vi "Flat.vi"(0 "Vin SMU":refnum<k15>, 1 "Input Voltage":dbl caption="voltage level" format="%.6p", 2 "Load current mA":dbl[](array[numeric]) caption="voltage level" format="%.6p", 5 "Load SMU":refnum<k15>, 7 "Vin DMM":refnum<k15>, 9 "Load DMM":refnum<k15>, 11 "error in (no error)":errorcluster) -> (4 "Load Regulation Ohm":dbl, 6 "Load Regulation %":dbl, 8 "output cluster":T1, 15 "error out":errorcluster)   [LabVIEW 2020]
uses:
  <instrlib>/niDCPower/nidcpower.llb/niDCPower Source Mode.ctl
  <instrlib>/niDCPower/nidcpower.llb/niDCPower Output Function.ctl
panel:
  in  "Nominal Voltage":dbl
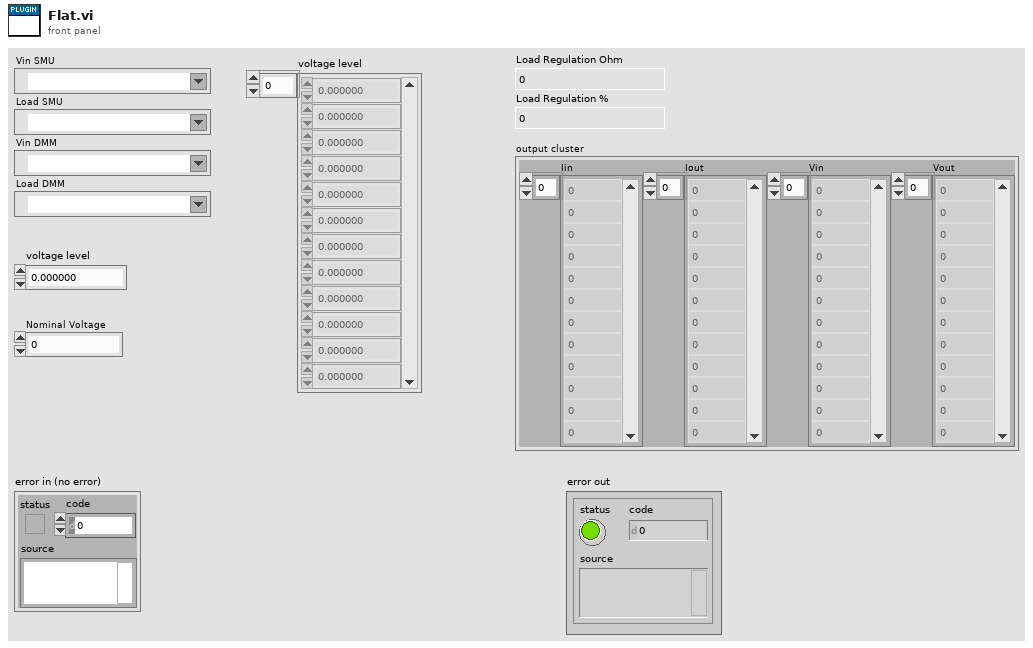
[diagram p1: front panel]
types:
  T1 = cluster{"Iin":dbl[], "Iout":dbl[], "Vin":dbl[], "Vout":dbl[]}
  T2 = typedef "niDCPower Output Function.ctl" = i32
  T3 = typedef "niDCPower Source Mode.ctl" = i32
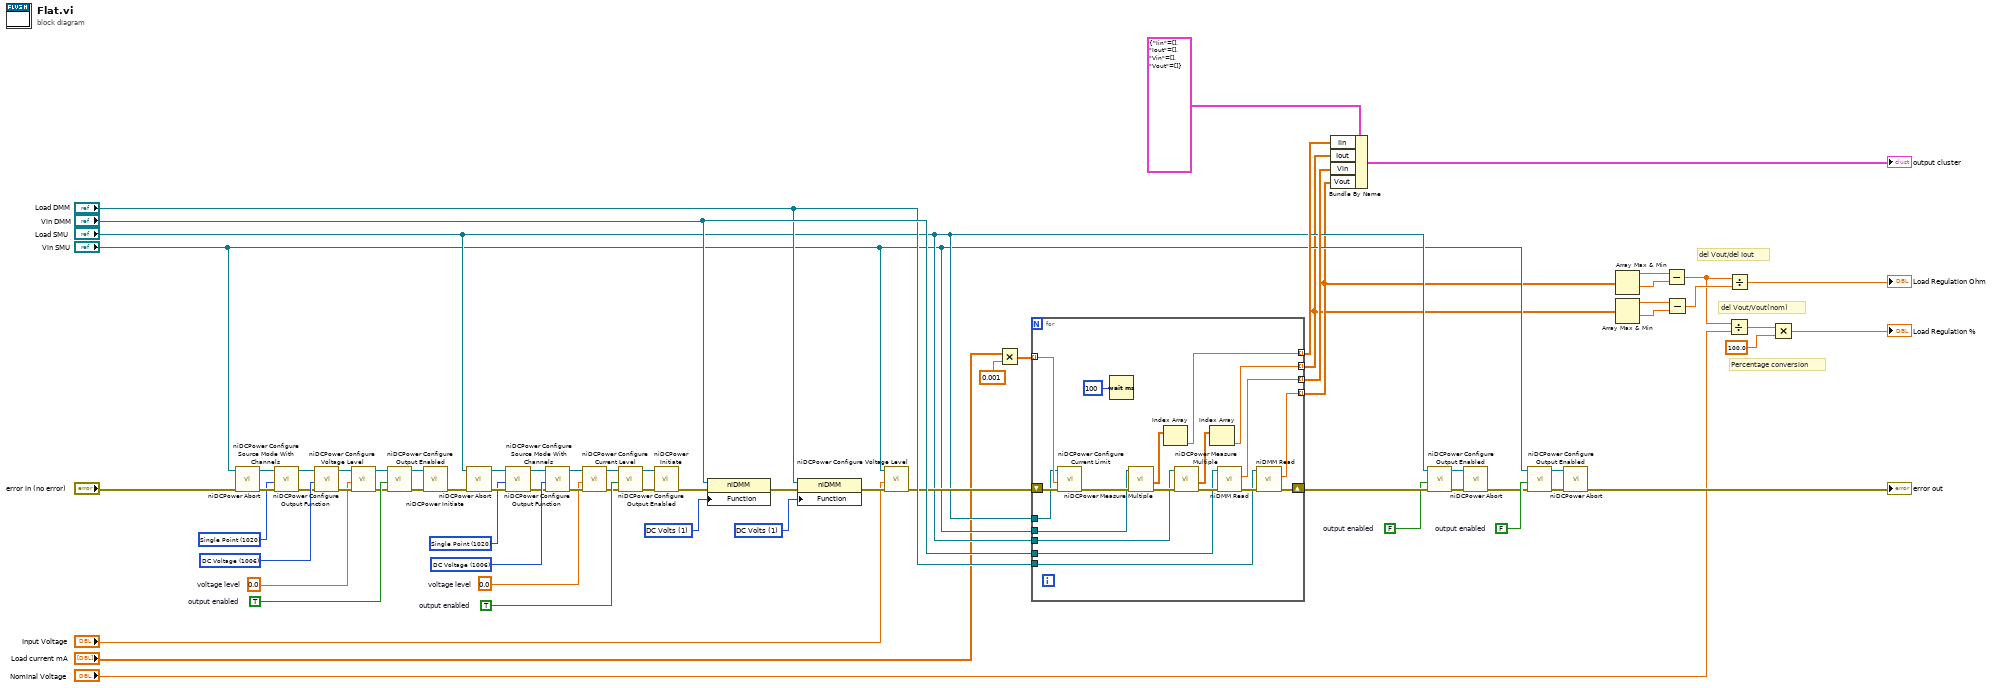
[diagram p0: block diagram]
diagram:
  w25 = FALSE  # output enabled
  w26 = FALSE  # output enabled
  w38 = 1 items=["DC Volts"=1, "AC Volts"=2, "DC Current"=3, "AC Current"=4, "2-Wire Resistance"=5, "4-Wire Resistance"=101, "Frequency"=104, "Period"=105, "AC Volts DC Coupled"=1001, "Diode"=1002, "Waveform Voltage"=1003, "Waveform Current"=1004, "Capacitance"=1005, "Inductance"=1006, "Temperature"=108] ("Configuration:Function")
  w39 = 1 items=["DC Volts"=1, "AC Volts"=2, "DC Current"=3, "AC Current"=4, "2-Wire Resistance"=5, "4-Wire Resistance"=101, "Frequency"=104, "Period"=105, "AC Volts DC Coupled"=1001, "Diode"=1002, "Waveform Voltage"=1003, "Waveform Current"=1004, "Capacitance"=1005, "Inductance"=1006, "Temperature"=108] ("Configuration:Function")
  w43 = 0.0  # voltage level
  w48 = TRUE  # output enabled
  w54 = T2 1006 items=["DC Voltage"=1006, "DC Current"=1007, "Pulse Voltage"=1049, "Pulse Current"=1050] ("output function")
  w51 = T3 1020 items=["Single Point"=1020, "Sequence"=1021] ("source mode")
  w61 = TRUE  # output enabled
  w62 = 0.0  # voltage level
  w68 = T2 1006 items=["DC Voltage"=1006, "DC Current"=1007, "Pulse Voltage"=1049, "Pulse Current"=1050] ("output function")
  w65 = T3 1020 items=["Single Point"=1020, "Sequence"=1021] ("source mode")
  # "del Vout/Vout(nom)"
  # "del Vout/del Iout"
  # "Percentage conversion"
  n1 = call <instrlib>:"niDCPower Abort.vi"("error in (no error)"="error in (no error)", "instrument handle"="Vin SMU") -> ("error out"=w69:errorcluster, "instrument handle out"=w70:refnum<k15>)  [unwired: 8 in]
  n2 = call <instrlib>:"niDCPower Configure Source Mode With Channels.vi"("error in (no error)"=w69, "source mode"=w65, "instrument handle"=w70) -> ("error out"=w67:errorcluster, "instrument handle out"=w66:refnum<k15>)  [unwired: 7 in]
  n3 = call <instrlib>:"niDCPower Configure Output Function.vi"("error in (no error)"=w67, "output function"=w68, "instrument handle"=w66) -> ("error out"=w64:errorcluster, "instrument handle out"=w63:refnum<k15>)  [unwired: 7 in]
  n4 = call <instrlib>:"niDCPower Configure Voltage Level.vi"("error in (no error)"=w64, "voltage level"=w62, "instrument handle"=w63) -> ("error out"=w60:errorcluster, "instrument handle out"=w57:refnum<k15>)  [unwired: 7 in]
  n5 = call <instrlib>:"niDCPower Configure Output Enabled.vi"("error in (no error)"=w60, "output enabled"=w61, "instrument handle"=w57) -> ("error out"=w59:errorcluster, "instrument handle out"=w58:refnum<k15>)  [unwired: 7 in]
  n6 = call <instrlib>:"niDCPower Initiate.vi"("error in (no error)"=w59, "instrument handle"=w58) -> ("error out"=w42:errorcluster)  [unwired: 8 in, 1 out]
  n7 = call <instrlib>:"niDCPower Abort.vi"("error in (no error)"=w42, "instrument handle"="Load SMU") -> ("error out"=w55:errorcluster, "instrument handle out"=w56:refnum<k15>)  [unwired: 8 in]
  n8 = call <instrlib>:"niDCPower Configure Source Mode With Channels.vi"("error in (no error)"=w55, "source mode"=w51, "instrument handle"=w56) -> ("error out"=w53:errorcluster, "instrument handle out"=w52:refnum<k15>)  [unwired: 7 in]
  n9 = call <instrlib>:"niDCPower Configure Output Function.vi"("error in (no error)"=w53, "output function"=w54, "instrument handle"=w52) -> ("error out"=w50:errorcluster, "instrument handle out"=w49:refnum<k15>)  [unwired: 7 in]
  n10 = call <instrlib>:"niDCPower Configure Current Level.vi"("error in (no error)"=w50, "current level"=w43, "instrument handle"=w49) -> ("error out"=w47:errorcluster, "instrument handle out"=w44:refnum<k15>)  [unwired: 7 in]
  n11 = call <instrlib>:"niDCPower Configure Output Enabled.vi"("error in (no error)"=w47, "output enabled"=w48, "instrument handle"=w44) -> ("error out"=w46:errorcluster, "instrument handle out"=w45:refnum<k15>)  [unwired: 7 in]
  n12 = call <instrlib>:"niDCPower Initiate.vi"("error in (no error)"=w46, "instrument handle"=w45) -> ("error out"=w40:errorcluster)  [unwired: 8 in, 1 out]
  n13 = property class="niDMM"(reference="Vin DMM", error in=w40, "Function"=w39) -> (error out=w37:errorcluster)  [unwired: 1 out]
  n14 = property class="niDMM"(reference="Load DMM", error in=w37, "Function"=w38) -> (error out=w36:errorcluster)  [unwired: 1 out]
  n15 = call <instrlib>:"niDCPower Configure Voltage Level.vi"("error in (no error)"=w36, "voltage level"="Input Voltage", "instrument handle"="Vin SMU") -> ("error out"=w28:errorcluster)  [unwired: 7 in, 1 out]
  n16 = Multiply(x="Load current mA", y=0.001 ("-x")) -> (x*y=w32:dbl[])
  n17 = for {
    shift-right: [w71] -> w27
    shift-left: w28 -> [w89]
    tunnel: [w84] -> w4 mode=indexing
    tunnel: [w82] -> w33 mode=indexing
    tunnel: [w80] -> w3 mode=indexing
    tunnel: [w85] -> w34 mode=indexing
    tunnel: w32 -> [w88] mode=indexing
    tunnel: "Load SMU" -> [w77]
    tunnel: "Vin SMU" -> [w76]
    tunnel: "Load SMU" -> [w75]
    tunnel: "Vin DMM" -> [w74]
    tunnel: "Load DMM" -> [w73]
    n18 = call <instrlib>:"niDCPower Configure Current Limit.vi"("error in (no error)"=w89, "current limit"=w88, "instrument handle"=w77) -> ("error out"=w86:errorcluster)  [unwired: 7 in, 1 out]
    n19 = Wait (ms)(milliseconds to wait=u32 100) -> ()  [unwired: 1 out]
    n20 = call <instrlib>:"niDCPower Measure Multiple.vi"("error in (no error)"=w86, "instrument handle"=w76) -> ("error out"=w79:errorcluster, "current measurements"=w87:dbl[])  [unwired: 6 in, 2 out]
    n21 = Index Array(array=w87) -> (element=w85:dbl)  [unwired: 1 in]
    n22 = call <instrlib>:"niDCPower Measure Multiple.vi"("error in (no error)"=w79, "instrument handle"=w75) -> ("error out"=w78:errorcluster, "current measurements"=w81:dbl[])  [unwired: 6 in, 2 out]
    n23 = Index Array(array=w81) -> (element=w80:dbl)  [unwired: 1 in]
    n24 = call <instrlib>:"niDMM Read.vi"("error in (no error)"=w78, "instrument handle"=w74) -> ("error out"=w83:errorcluster, "Measurement"=w82:dbl)  [unwired: 7 in, 1 out]
    n25 = call <instrlib>:"niDMM Read.vi"("error in (no error)"=w83, "instrument handle"=w73) -> ("error out"=w71:errorcluster, "Measurement"=w84:dbl)  [unwired: 7 in, 1 out]
  }
  n26 = Bundle By Name(cluster=T1 {"Iin"=[], "Iout"=[], "Vin"=[], "Vout"=[]}, "Iin"=w34, "Iout"=w3, "Vin"=w33, "Vout"=w4) -> (→"output cluster":T1)
  n27 = call <instrlib>:"niDCPower Configure Output Enabled.vi"("error in (no error)"=w27, "output enabled"=w26, "instrument handle"="Load SMU") -> ("error out"=w22:errorcluster, "instrument handle out"=w21:refnum<k15>)  [unwired: 7 in]
  n28 = call <instrlib>:"niDCPower Abort.vi"("error in (no error)"=w22, "instrument handle"=w21) -> ("error out"=w18:errorcluster)  [unwired: 8 in, 1 out]
  n29 = call <instrlib>:"niDCPower Configure Output Enabled.vi"("error in (no error)"=w18, "output enabled"=w25, "instrument handle"="Vin SMU") -> ("error out"=w24:errorcluster, "instrument handle out"=w23:refnum<k15>)  [unwired: 7 in]
  n30 = call <instrlib>:"niDCPower Abort.vi"("error in (no error)"=w24, "instrument handle"=w23) -> ("error out"=→"error out":errorcluster)  [unwired: 8 in, 1 out]
  n31 = Array Max & Min(array=w4) -> (max value=w16:dbl, min value=w7:dbl)  [unwired: 2 out]
  n32 = Array Max & Min(array=w3) -> (max value=w15:dbl, min value=w14:dbl)  [unwired: 2 out]
  n33 = Subtract(x=w16, y=w7) -> (x-y=w8:dbl)
  n34 = Subtract(x=w15, y=w14) -> (x-y=w13:dbl)
  n35 = Divide(x=w8, y="Nominal Voltage") -> (x/y=w11:dbl)
  n36 = Divide(x=w8, y=w13) -> (x/y=→"Load Regulation Ohm":dbl)
  n37 = Multiply(x=w11, y=100.0) -> (x*y=→"Load Regulation %":dbl)
